vi "Rotate (Greyscale).vi"(4 "Border Colour (Default: 0)":u8, 5 "Boarder Type (Default: DEFAULT)":T2=enum."DEFAULT", 6 "Destination Sizing Mode (Default: Resize)":T1, 7 "Interpolation Mode (Default: CUBIC)":T4=enum."CUBIC", 8 "error in (no error)":errorcluster, 9 "Rotation (Deg)":dbl, 10 "Greyscale Destination Image in":T3, 11 "Greyscale Source Image in":T3) -> (0 "error out":errorcluster, 3 "Greyscale Destination Image":T3)   [LabVIEW 2020, in "image.lvlib"]
doc: "Rotate the Source Image by the specified number of degrees. Use the \"Destination Sizing Mode\" input to control how the Destination Image will be sized to fit."
uses:
  image.lvlib
  Greyscale Image.ctl
  Interpolation Mode.ctl
  Border Type.ctl
  Destination Sizing Mode.ctl
  6b7c46c8-7bec-461b-8321-5c3565ab93c7.vi
  <vilib>/Utility/error.llb/Error Cluster From Error Code.vi
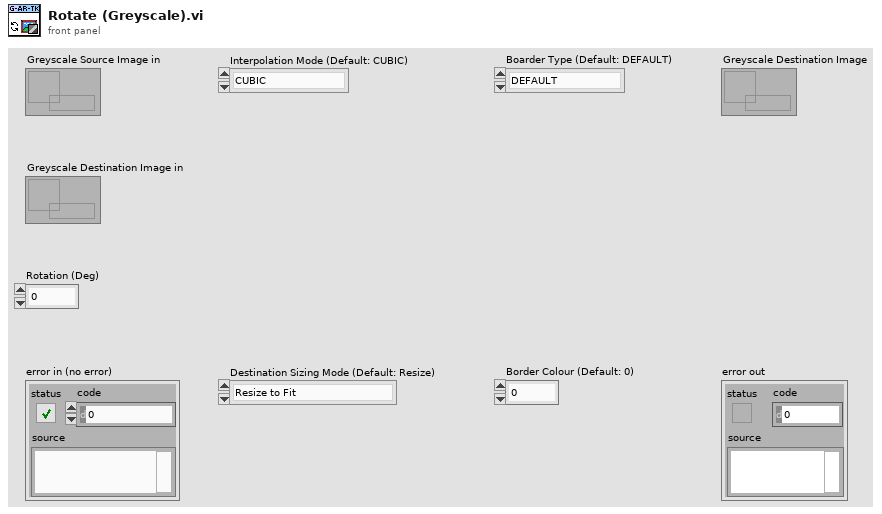
[diagram p1: front panel]
types:
  T1 = typedef "image.lvlib/Destination Sizing Mode.ctl" = enum8{"Resize to Fit", "Use Source Image Size"}
  T2 = typedef "image.lvlib/Border Type.ctl" = enum8{"CONSTANT", "REPLICATE", "REFLECT", "WRAP", "TRANSPARENT", "DEFAULT", "ISOLATED"}
  T3 = typedef "image.lvlib/Greyscale Image.ctl" = refnum<data-value>
  T4 = typedef "image.lvlib/Interpolation Mode.ctl" = enum8{"NEAREST", "LINEAR", "CUBIC", "AREA", "LANCZOS", "LINEAR_EXACT", "NEAREST_EXACT", "MAX"}
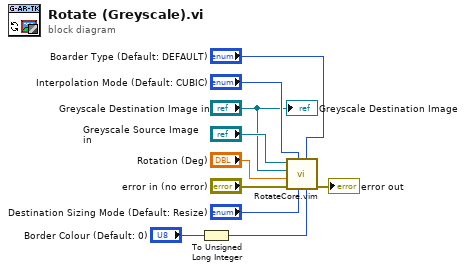
[diagram p0: block diagram]
diagram:
  n1 = To Unsigned Long Integer(number="Border Colour (Default: 0)") -> (unsigned 32bit integer=w8:u32)
  n2 = call "RotateCore.vim"("Border Colour"=w8, "Boarder Type"="Boarder Type (Default: DEFAULT)", "Destination Sizing Mode (Default: Resize)"="Destination Sizing Mode (Default: Resize)", "Interpolation Mode"="Interpolation Mode (Default: CUBIC)", "error in (no error)"="error in (no error)", "Rotation"="Rotation (Deg)", "Dst"="Greyscale Destination Image in", "Src"="Greyscale Source Image in") -> ("error out"=→"error out":errorcluster)  [unwired: 3 in]
  "Greyscale Destination Image" <- "Greyscale Destination Image in"
